vi "CLSUIP_SetControlInformation.vi"(8 "error in (no error)":errorcluster, 10 "Control Information":T1, 11 "Ctl Refnum":refnum<vi>) -> (0 "error out":errorcluster, 3 "Ctl Refnum out":refnum<vi>)   [LabVIEW 2021, in "MemberVICreation.lvlib"]
uses:
  <resource>/Framework/Providers/LVClassLibrary/NewAccessors/MemberVICreation.lvlib
  <resource>/Framework/Providers/LVClassLibrary/NewAccessors/CLSUIP_ControlInformation.ctl
  <vilib>/Utility/miscctls.llb/LVPositionTypeDef.ctl
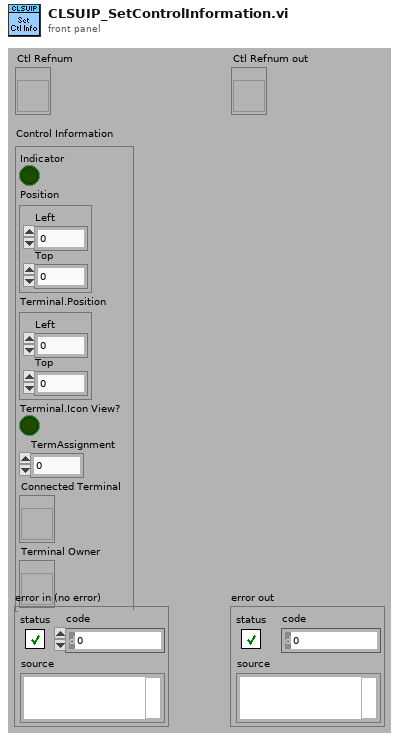
[diagram p1: front panel]
types:
  T1 = typedef "MemberVICreation.lvlib/CLSUIP_ControlInformation.ctl" = cluster{"Indicator":bool, "Position":T2, "Terminal.Position":T2, "Terminal.Icon View?":bool, "TermAssignment":i32, "Connected Terminal":refnum<vi>, "Terminal Owner":refnum<vi>}
  T2 = typedef "LVPositionTypeDef.ctl" = cluster{"Left":i32, "Top":i32}
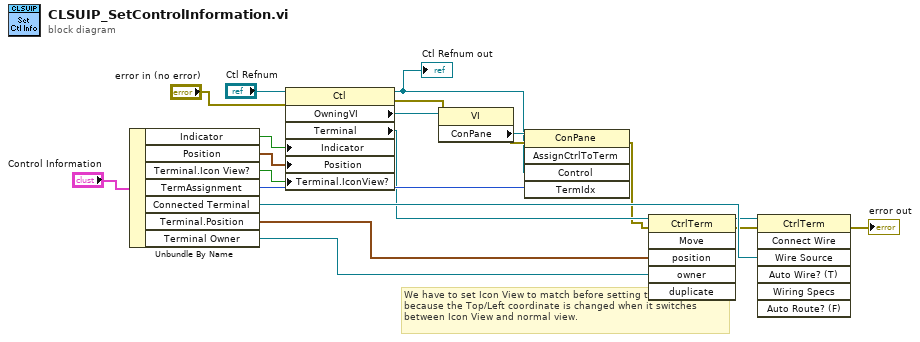
[diagram p0: block diagram]
diagram:
  # "We have to set Icon View to match before setting the position\nbecause the Top/Left coordinate is changed when it switches\nbetween Icon View and normal view."
  n1 = Unbundle By Name("Control Information") -> ("Indicator"=w16:bool, "Position"=w15:T2, "Terminal.Icon View?"=w14:bool, "TermAssignment"=w10:i32, "Connected Terminal"=w9:refnum<vi>, "Terminal.Position"=w2:T2, "Terminal Owner"=w1:refnum<vi>)
  n2 = property class="Ctl"(reference="Ctl Refnum", error in="error in (no error)", "Indicator"=w16, "Position"=w15, "Terminal.IconView?"=w14) -> (reference out=w11:refnum<vi>, error out=w8:errorcluster, "OwningVI"=w19:refnum<vi>, "Terminal"=w4:refnum<vi>)
  "Ctl Refnum out" <- w11
  n3 = property class="VI"(reference=w19, error in=w8) -> (error out=w12:errorcluster, "ConPane"=w13:refnum<vi>)  [unwired: 1 out]
  n4 = invoke class="ConPane" method="AssignCtrlToTerm"(reference=w13, error in=w12, "Control"=w11, "TermIdx"=w10) -> (error out=w3:errorcluster)  [unwired: 1 in, 4 out]
  n5 = invoke class="CtrlTerm" method="Move"(reference=w4, error in=w3, "position"=w2, "owner"=w1) -> (reference out=w6:refnum<vi>, error out=w5:errorcluster)  [unwired: 2 in, 4 out]
  n6 = invoke class="CtrlTerm" method="Connect Wire"(reference=w6, error in=w5, "Wire Source"=w9) -> (error out=→"error out":errorcluster)  [unwired: 4 in, 6 out]
